vi "dump.vi"(8 "error in (no error)":errorcluster, 10 "indent":T1, 11 "OpResult in":refnum<class "OpResult.lvclass">) -> (0 "error out":errorcluster, 2 "mlir":string, 3 "OpResult out":refnum<class "OpResult.lvclass">)   [LabVIEW 2020, in "mlir.lvlib" / "OpResult.lvclass"]
uses:
  OpResult.lvclass
  Node/indent.ctl
  OpResult.lvclass/OpResult.ctl
  21ecda14-79e2-460a-a8ba-59f7a8533e5a.vi
  <userlib>/_OpenG.lib/string/string.llb/Format Variant Into String__ogtk.vi
  SsaId/SsaId.lvclass
  mlir.lvlib
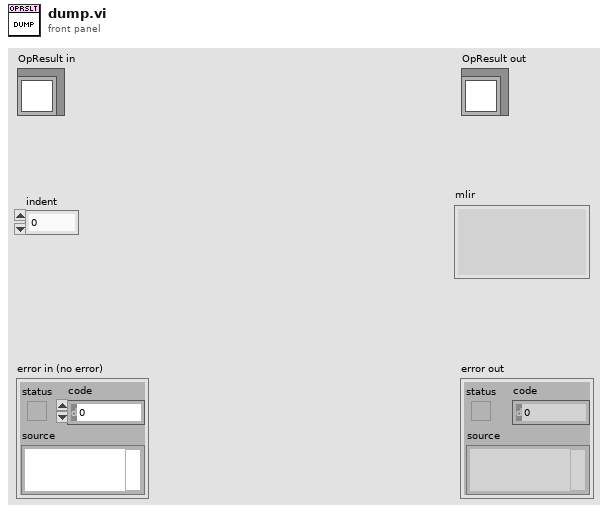
[diagram p1: front panel]
types:
  T1 = typedef "mlir.lvlib/indent.ctl" = u32
  T2 = typedef "mlir.lvlib/OpResult.lvclass/count.ctl" = u32
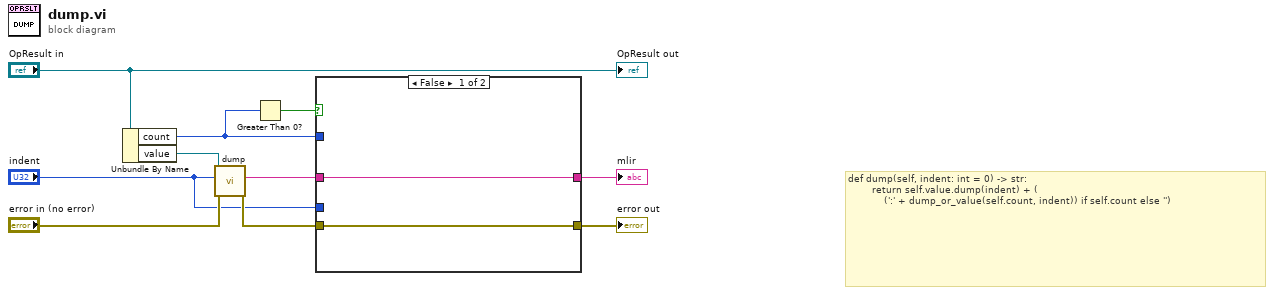
[diagram p0: block diagram]
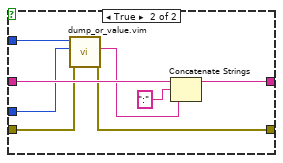
[diagram p2: hidden frame]
diagram:
  # "def dump(self, indent: int = 0) -> str:\n        return self.value.dump(indent) + (\n            (':' + dump_or_value(self.count, indent)) if self.count else '')"
  n1 = Unbundle By Name("OpResult in") -> ("count"=w7:T2, "value"=w10:refnum<class "SsaId.lvclass">)
  n2 = call-dynamic "dump.vi"("error in (no error)"="error in (no error)", "indent"="indent", "SsaId in"=w10) -> ("error out"=w4:errorcluster, "mlir"=w8:string)  [unwired: 6 in, 1 out]
  n3 = Greater Than 0?(x=w7) -> (x > 0?=w9:bool)
  n4 = case shown="False" w9 {
    tunnel: w8 -> [w12 w20]
    tunnel: w7 -> [_ w17]
    tunnel: [w12 w18] -> w6
    tunnel: w4 -> [w11 w16]
    tunnel: [w11 w15] -> w3
    tunnel: "indent" -> [_ w13]
    frame False {
    }
    frame True {
      n5 = call "dump_or_value.vim"("error in (no error)"=w16, "indent"=w13, "value"=w17) -> ("error out"=w15:errorcluster, "mlir"=w14:string)  [unwired: 7 in]
      n6 = Concatenate Strings(w20, ":" ("string"), w14) -> (w18:string)
    }
  }
  "error out" <- w3
  "mlir" <- w6
  "OpResult out" <- "OpResult in"
